vi "시리얼_닫기.vi"(8 "Error In":errorcluster caption="에러 입력", 11 "VISA 리소스 이름":refnum<visa-resource-name>) -> (0 "Error Out":errorcluster caption="에러 출력")   [LabVIEW 2018]
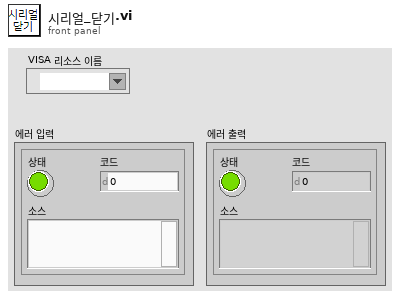
[diagram p1: front panel]
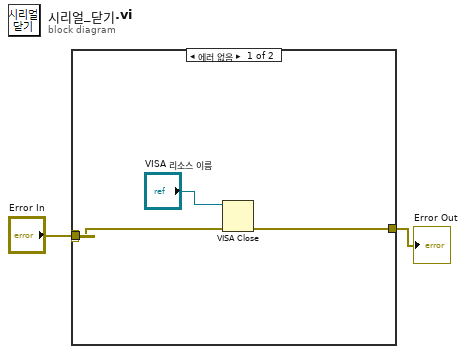
[diagram p0: block diagram]
diagram:
  n1 = case shown="에러 없음" "Error In" {
    selector: "Error In" -> [w5 w6]
    tunnel: [_ w6] -> _
    tunnel: [w4 _] -> w1
    frame No Error {
      n2 = VISA Close(VISA resource name="VISA 리소스 이름", error in (no error)=w5) -> (error out=w4:errorcluster)
    }
    frame Error {
    }
  }
  "Error Out" <- w1
